vi "practice5(経過時間).vi"() -> ()   [LabVIEW 2018]
panel:
  out "文字列":string
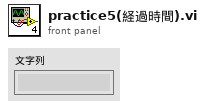
[diagram p1: front panel]
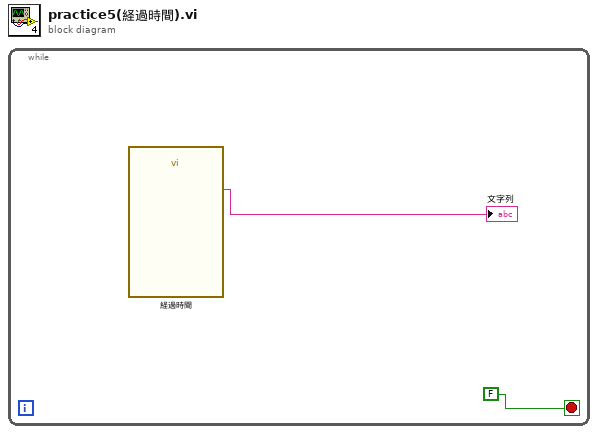
[diagram p0: block diagram]
diagram:
  n1 = while {
    stop <- FALSE stop-if-true
    n2 = call "経過時間"() -> ("Elapsed Time Text"=→"文字列":string)  [unwired: 12 in, 7 out]
  }
